vi "速度转换.vi"(11 "In":sgl) -> (3 "Out":sgl format="%#_6f")   [LabVIEW 2020, in "输出轴伺服.lvlib"]
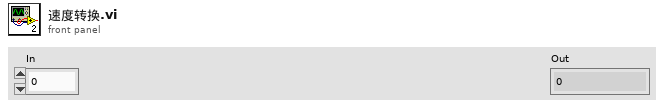
[diagram p1: front panel]
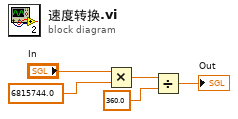
[diagram p0: block diagram]
diagram:
  n1 = Multiply(x="In", y=sgl 6815744.0) -> (x*y=w4:sgl)
  n2 = Divide(x=w4, y=sgl 360.0) -> (x/y=→"Out":sgl)
